vi "errorMessage.vi"(0 "messageText":string) -> (1 "Window Handle out":T2 items=["HWND_TOP"=0, "HWND_BOTTOM"=1, "HWND_TOPMOST"=-1, "HWND_NOTOPMOST"=-2], 2 "Message Box Button":T1, 3 "Timeout":bool)   [LabVIEW 2015]
uses:
  C:/Users/sims01/Downloads/AIT - WinAPI - MessageBoxTimeout/Support/AIT - WinAPI - Window Handle.ctl
  C:/Users/sims01/Downloads/AIT - WinAPI - MessageBoxTimeout/Support/Constants/Support/AIT - WinAPI - Message Box Button.ctl
  C:/Users/sims01/Downloads/AIT - WinAPI - MessageBoxTimeout/Support/Constants/Support/AIT - WinAPI - Message Box Type.ctl
  C:/Users/sims01/Downloads/AIT - WinAPI - MessageBoxTimeout/Support/Constants/Support/AIT - WinAPI - Message Box Icon.ctl
  C:/Users/sims01/Downloads/AIT - WinAPI - MessageBoxTimeout/Support/Constants/Support/AIT - WinAPI - Message Box Default Button.ctl
  C:/Users/sims01/Downloads/AIT - WinAPI - MessageBoxTimeout/Support/Constants/Support/AIT - WinAPI - Message Box Modality.ctl
  C:/Users/sims01/Downloads/AIT - WinAPI - MessageBoxTimeout/Support/Constants/Support/AIT - WinAPI - Message Box Misc Setting.ctl
  C:/Users/sims01/Downloads/AIT - WinAPI - MessageBoxTimeout/Support/Constants/Support/AIT - WinAPI - LanguageId.ctl
  C:/Users/sims01/Downloads/AIT - WinAPI - MessageBoxTimeout/Support/Constants/Support/AIT - WinAPI - Message Box Misc Settings (Multiple).vi
  user32.dll
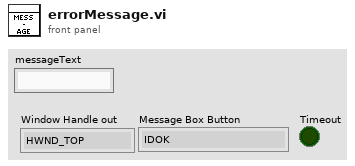
[diagram p1: front panel]
types:
  T1 = typedef "AIT - WinAPI - Message Box Button.ctl" = enum16{"IDOK", "IDCANCEL", "IDABORT", "IDRETRY", "IDIGNORE", "IDYES", "IDNO", "IDTRYAGAIN", "IDCONTINUE", "MB_TIMEDOUT"}
  T2 = typedef "AIT - WinAPI - Window Handle.ctl" = i32
  T3 = typedef "AIT - WinAPI - Message Box Type.ctl" = enum16{"MB_ABORTRETRYIGNORE", "MB_CANCELTRYCONTINUE", "MB_HELP", "MB_OK", "MB_OKCANCEL", "MB_RETRYCANCEL", "MB_YESNO", "MB_YESNOCANCEL"}
  T4 = typedef "AIT - WinAPI - Message Box Icon.ctl" = enum16{"NONE", "MB_ICONEXCLAMATION", "MB_ICONWARNING", "MB_ICONINFORMATION", "MB_ICONASTERISK", "MB_ICONQUESTION", "MB_ICONSTOP", "MB_ICONERROR", "MB_ICONHAND"}
  T5 = typedef "AIT - WinAPI - Message Box Default Button.ctl" = enum16{"MB_DEFBUTTON1", "MB_DEFBUTTON2", "MB_DEFBUTTON3", "MB_DEFBUTTON4"}
  T6 = typedef "AIT - WinAPI - Message Box Modality.ctl" = enum16{"MB_APPLMODAL", "MB_SYSTEMMODAL", "MB_TASKMODAL"}
  T7 = typedef "AIT - WinAPI - Message Box Misc Setting.ctl" = enum16{"MB_DEFAULT_DESKTOP_ONLY", "MB_RIGHT", "MB_RTLREADING", "MB_SETFOREGROUND", "MB_TOPMOST", "MB_SERVICE_NOTIFICATION", "MB_SERVICE_NOTIFICATION_NT3X"}
  T8 = typedef "AIT - WinAPI - LanguageId.ctl" = enum16{"wdAfrikaans", "wdAlbanian", "wdAmharic", "wdArabic", "wdArabicAlgeria", "wdArabicBahrain", "wdArabicEgypt", "wdArabicIraq", "wdArabicJordan", "wdArabicKuwait", "wdArabicLebanon", "wdArabicLibya", "wdArabicMorocco", "wdArabicOman", "wdArabicQatar", "wdArabicSyria", "wdArabicTunisia", "wdArabicUAE", "wdArabicYemen", "wdArmenian", "wdAssamese", "wdAzeriCyrillic", "wdAzeriLatin", "wdBasque", "wdBelgianDutch", "wdBelgianFrench", "wdBengali", "wdBrazilianPortuguese", "wdBulgarian", "wdBurmese", "wdByelorussian", "wdCatalan", "wdCherokee", "wdChineseHongKongSAR", "wdChineseMacaoSAR", "wdChineseSingapore", "wdCroatian", "wdCzech", "wdDanish", "wdDivehi", "wdDutch", "wdDzongkhaBhutan", "wdEdo", "wdEnglishAUS", "wdEnglishBelize", "wdEnglishCanadian", "wdEnglishCaribbean", "wdEnglishIndonesia", "wdEnglishIreland", "wdEnglishJamaica", "wdEnglishNewZealand", "wdEnglishPhilippines", "wdEnglishSouthAfrica", "wdEnglishTrinidadTobago", "wdEnglishUK", "wdEnglishUS", "wdEnglishZimbabwe", "wdEstonian", "wdFaeroese", "wdFarsi", "wdFilipino", "wdFinnish", "wdFrench", "wdFrenchCameroon", "wdFrenchCanadian", "wdFrenchCotedIvoire", "wdFrenchHaiti", "wdFrenchLuxembourg", "wdFrenchMali", "wdFrenchMonaco", "wdFrenchMorocco", "wdFrenchReunion", "wdFrenchSenegal", "wdFrenchWestIndies", "wdFrenchZaire", "wdFrisianNetherlands", "wdFulfulde", "wdGaelicIreland", "wdGaelicScotland", "wdGalician", "wdGeorgian", "wdGerman", "wdGermanAustria", "wdGermanLiechtenstein", "wdGermanLuxembourg", "wdGreek", "wdGuarani", "wdGujarati", "wdHausa", "wdHawaiian", "wdHebrew", "wdHindi", "wdHungarian", "wdIbibio", "wdIcelandic", "wdIgbo", "wdIndonesian", "wdInuktitut", "wdItalian", "wdJapanese", "wdKannada", "wdKanuri", "wdKashmiri", "wdKazakh", "wdKhmer", "wdKirghiz", "wdKonkani", "wdKorean", "wdKyrgyz", "wdLanguageNone", "wdLao", "wdLatin", "wdLatvian", "wdLithuanian", "wdMacedonian", "wdMalayalam", "wdMalayBruneiDarussalam", "wdMalaysian", "wdMaltese", "wdManipuri", "wdMarathi", "wdMexicanSpanish", "wdMongolian", "wdNepali", "wdNoProofing", "wdNorwegianBokmol", "wdNorwegianNynorsk", "wdOriya", "wdOromo", "wdPashto", "wdPolish", "wdPortuguese", "wdPunjabi", "wdRhaetoRomanic", "wdRomanian", "wdRomanianMoldova", "wdRussian", "wdRussianMoldova", "wdSamiLappish", "wdSanskrit", "wdSerbianCyrillic", "wdSerbianLatin", "wdSesotho", "wdSimplifiedChinese", "wdSindhi", "wdSindhiPakistan", "wdSinhalese", "wdSlovak", "wdSlovenian", "wdSomali", "wdSorbian", "wdSpanish", "wdSpanishArgentina", "wdSpanishBolivia", "wdSpanishChile", "wdSpanishColombia", "wdSpanishCostaRica", "wdSpanishDominicanRepublic", "wdSpanishEcuador", "wdSpanishElSalvador", "wdSpanishGuatemala", "wdSpanishHonduras", "wdSpanishModernSort", "wdSpanishNicaragua", "wdSpanishPanama", "wdSpanishParaguay", "wdSpanishPeru", "wdSpanishPuertoRico", "wdSpanishUruguay", "wdSpanishVenezuela", "wdSutu", "wdSwahili", "wdSwedish", "wdSwedishFinland", "wdSwissFrench", "wdSwissGerman", "wdSwissItalian", "wdSyriac", "wdTajik", "wdTamazight", "wdTamazightLatin", "wdTamil", "wdTatar", "wdTelugu", "wdThai", "wdTibetan", "wdTigrignaEritrea", "wdTigrignaEthiopic", "wdTraditionalChinese", "wdTsonga", "wdTswana", "wdTurkish", "wdTurkmen", "wdUkrainian", "wdUrdu", "wdUzbekCyrillic", "wdUzbekLatin", "wdVenda", "wdVietnamese", "wdWelsh", "wdXhosa", "wdYi", "wdYiddish", "wdYoruba", "wdZulu"}
  T9 = cluster{"Message Box Type":T3, "Message Box Icon":T4, "Message Box Default Button":T5, "Message Box Modality":T6, "Message Box Misc Settings":T7[], "LanguageId":T8}
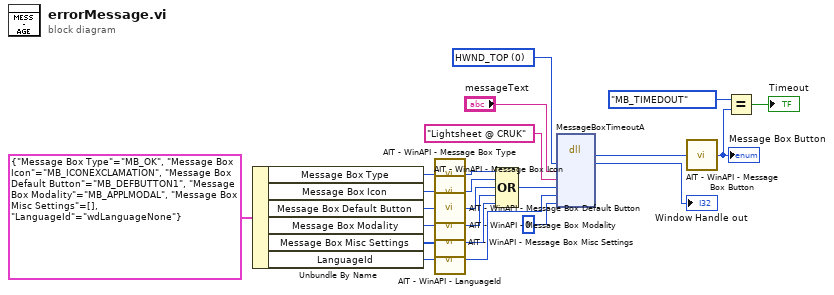
[diagram p0: block diagram]
diagram:
  w8 = T2 0 items=["HWND_TOP"=0, "HWND_BOTTOM"=1, "HWND_TOPMOST"=-1, "HWND_NOTOPMOST"=-2] ("Window Handle in")
  n1 = Unbundle By Name(T9 {"Message Box Type"=enum."MB_OK", "Message Box Icon"=enum."MB_ICONEXCLAMATION", "Message Box Default Button"=enum."MB_DEFBUTTON1", "Message Box Modality"=enum."MB_APPLMODAL", "Message Box Misc Settings"=[], "LanguageId"=enum."wdLanguageNone"} ("MessageBox Settings")) -> ("Message Box Type"=w21:T3, "Message Box Icon"=w20:T4, "Message Box Default Button"=w18:T5, "Message Box Modality"=w19:T6, "Message Box Misc Settings"=w22:T7[], "LanguageId"=w23:T8)
  n2 = call "AIT - WinAPI - Message Box Type.vi"("Message Box Type"=w21) -> ("Message Box Type"=w12:u32)  [unwired: 4 out]
  n3 = call "AIT - WinAPI - Message Box Icon.vi"("Message Box Icon"=w20) -> ("Message Box Icon"=w11:u32)  [unwired: 4 out]
  n4 = call "AIT - WinAPI - Message Box Default Button.vi"("Message Box Default Button"=w18) -> ("Message Box Default Button"=w10:u32)  [unwired: 4 out]
  n5 = call "AIT - WinAPI - Message Box Modality.vi"("Message Box Modality"=w19) -> ("Message Box Modality"=w13:u32)  [unwired: 4 out]
  n6 = call-poly "AIT - WinAPI - Message Box Misc Settings.vi"("Message Box Misc Setting"=w22) -> ("Message Box Misc Setting"=w14:u32)  [unwired: 4 out]
  n7 = call "AIT - WinAPI - LanguageId.vi"("LanguageId"=w23) -> ("Message Box Icon"=w15:i32)  [unwired: 4 out]
  n8 = Compound Arithmetic op=OR(w12, w11, w10, w13, w14) -> (w17:u32)
  n9 = dll-call lib="user32.dll" fn="MessageBoxTimeoutA" label="MessageBoxTimeout"("hWnd"=w8, "lpText"="messageText", "lpCaption"="Lightsheet @ CRUK" ("Dialog Title Text"), "uType"=w17, "wLanguageId"=w15, "dwMilliseconds"=0 ("Timeout")) -> ("return type"=w9:i16, "hWnd"=→"Window Handle out":i32)  [unwired: 8 in, 2 out]
  n10 = call "AIT - WinAPI - Message Box Button.vi"("Message Box Button"=w9) -> ("Message Box Button"=w2:T1)  [unwired: 4 out]
  "Message Box Button" <- w2
  n11 = Equal?(x=AIT_-_WinAPI_-_Message_Box_Button."MB_TIMEDOUT" ("y"), y=w2) -> (x = y?=→"Timeout":bool)
